vi "readID_TCP.vi"() -> ()   [LabVIEW 2017]
panel:
  out "Numeric":i32
  out "x = y?":bool
  in  "substring 2":string="“\u0010\u0000$"
  out "substring":string
  in  "long":bool
  in  "数组 6":string[](array[string])=["shift:\u0005\u0000\u0000\u0000\u001f\u0000", "shift:\u0004\u0000\u0000\u0000\u0002\u0000", "shift: \u0000\u0000\u0000\u0000\u0000\u0000\u0000\u0000\u0000\u0000\u0000"]
  in  "数组 5":string[](array[string])=["shift: \u0000\u0000\u0000ÿÿÿÿ\u0000\u0000\u0000\u0000", "shift:(\u0000\u0000\u0000\u0002\u0000\u0000\u0000\u0000\u0000\u0000\u0000\u0000\u0000\u0000\u0000\u0000\u0000", "shift: \u0000\u0000\u0000\u0000\u0000\u0000\u0000\u0000\u0000\u0000\u0000"]
  out "k7 idcode":string
  out "sp6 idcode":string
  in  "数组 4":string[](array[string])=["settck:d\u0000\u0000\u0000"]
  in  "shift string":string="shift:\u0005\u0000\u0000\u0000\u001f\u0000"
  in  "数组 3":string[](array[string])=["shift:\u0005\u0000\u0000\u0000\u001f\u0000"]
  in  "停止":bool
  out "数值":i32=2
  out "数据输出":string
  in  "字符串 2":string="shift:\u0005\u0000\u0000\u001f\u0000"
  in  "字符串":string="getinfo:"
  in  "数组 2":string[](array[string])=["shift:\u0005\u0000\u0000\u0000\u001f\u0000", "shift:\u0004\u0000\u0000\u0000\u0002\u0000", "shift: \u0000\u0000\u0000\u0000\u0000\u0000\u0000\u0000\u0000\u0000\u0000"]
  out "错误输出":errorcluster
  in  "数组":string[](array[string])=["getinfo:"]
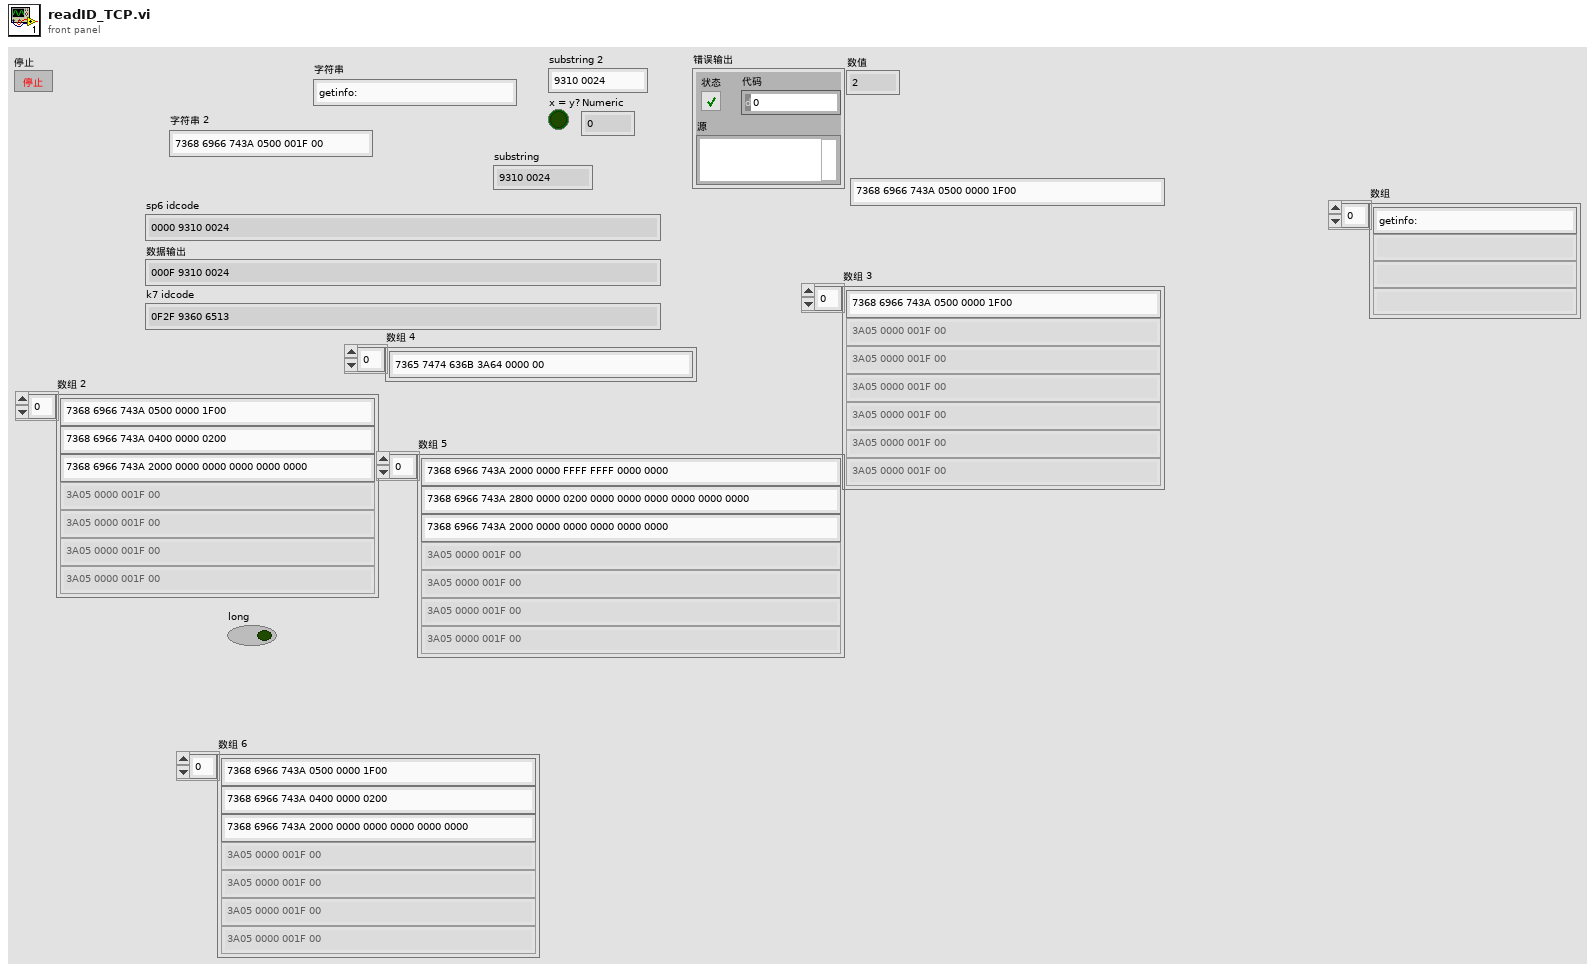
[diagram p1: front panel]
types:
  T1 = enum16{"Standard", "Buffered", "CRLF", "Immediate"}
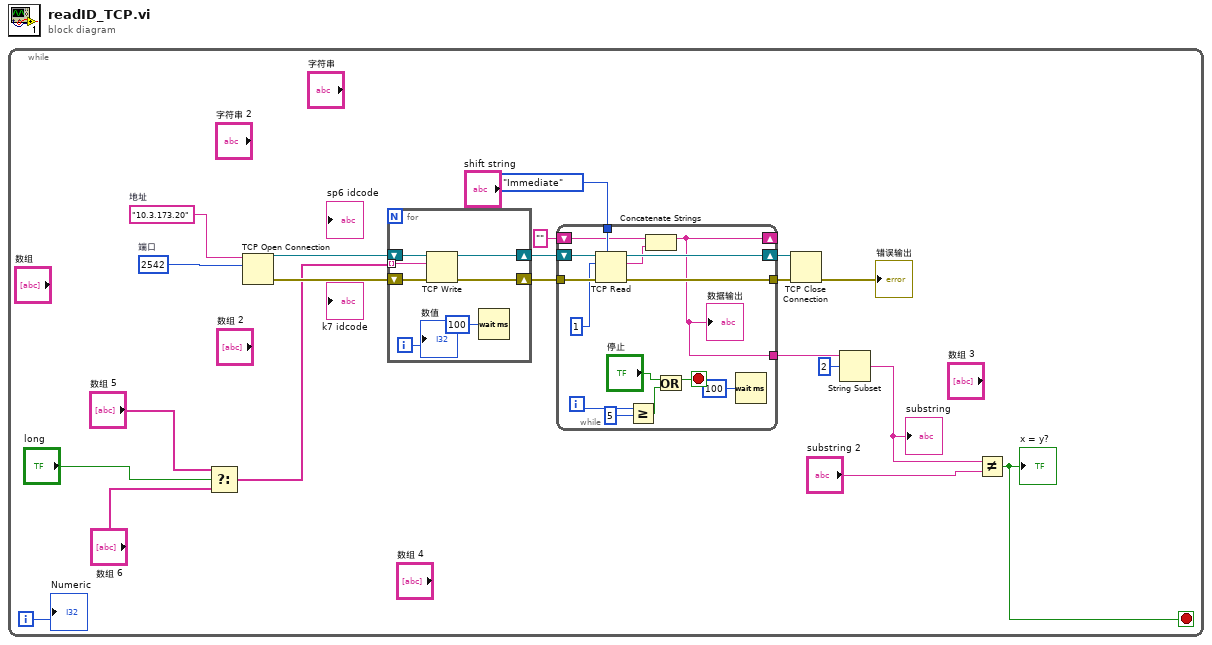
[diagram p0: block diagram]
diagram:
  n1 = while {
    i -> [w1]
    stop <- w2 stop-if-true
    w20 = u16 2542  # 端口
    w21 = "10.3.173.20"  # 地址
    n2 = Select(t="数组 5", s="long", f="数组 6") -> (s? t:f=w9:string[])
    n3 = TCP Open Connection(address=w21, remote port or service name=w20) -> (connection ID=w19:refnum<k5>, error out=w18:errorcluster)  [unwired: 3 in]
    n4 = for {
      shift-right: [w41] -> w17
      shift-left: w19 -> [w43]
      shift-right: [w40] -> w14
      shift-left: w18 -> [w42]
      tunnel: w9 -> [w39] mode=indexing
      i -> [w37]
      n5 = TCP Write(connection ID=w43, data in=w39, error in (no error)=w42) -> (connection ID out=w41:refnum<k5>, error out=w40:errorcluster)  [unwired: 1 in, 1 out]
      n6 = Wait (ms)(milliseconds to wait=u32 100) -> ()  [unwired: 1 out]
      "数值" <- w37
    }
    n7 = while {
      tunnel: T1."Immediate" ("模式（标准）") -> [w32]
      shift-right: [w35] -> w15
      shift-left: w17 -> [w36]
      shift-right: [w22] -> _
      shift-left: "" -> [w30]
      tunnel: w14 -> [w34]
      tunnel: [w33] -> w13
      tunnel: [w22] -> w6
      i -> [w26]
      stop <- w24 stop-if-true
      n8 = TCP Read(connection ID=w36, bytes to read=1 ("读取的字节"), error in (no error)=w34, 7:w32) -> (connection ID out=w35:refnum<k5>, data out=w29:string, error out=w33:errorcluster)  [unwired: 1 in]
      n9 = Greater Or Equal?(x=w26, y=5) -> (x >= y?=w23:bool)
      n10 = Concatenate Strings(w30, w29) -> (w22:string)
      "数据输出" <- w22
      n11 = Or(x="停止", y=w23) -> (x .or. y?=w24:bool)
      n12 = Wait (ms)(milliseconds to wait=u32 100) -> ()  [unwired: 1 out]
    }
    n13 = TCP Close Connection(connection ID=w15, error in (no error)=w13) -> (error out=→"错误输出":errorcluster)  [unwired: 1 in, 1 out]
    n14 = String Subset(string=w6, offset (0)=2) -> (substring=w3:string)  [unwired: 1 in]
    "substring" <- w3
    n15 = Not Equal?(x=w3, y="substring 2") -> (x != y?=w2:bool)
    "x = y?" <- w2
    "Numeric" <- w1
  }
